vi "Close.vi"(8 "error in":errorcluster, 11 "IMAQdx Triggered Continuous Acquisition in":refnum<class "IMAQdx Triggered Continuous Acquisition.lvclass">) -> (0 "error out":errorcluster, 3 "IMAQdx Triggered Continuous Acquisition out":refnum<class "IMAQdx Triggered Continuous Acquisition.lvclass">)   [LabVIEW 2024, in "IMAQdx Triggered Continuous Acquisition.lvclass"]
uses:
  IMAQdx Triggered Continuous Acquisition.lvclass
  IMAQdx Triggered Continuous Acquisition.lvclass/IMAQdx Triggered Continuous Acquisition.ctl
  Base/IMAQdx Base Configure Strategy.lvclass
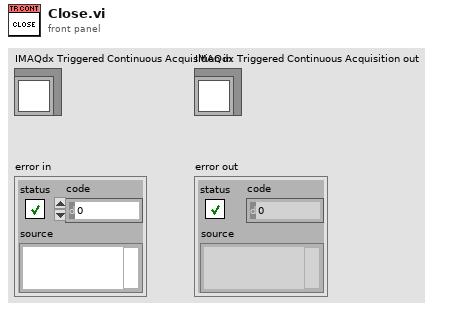
[diagram p1: front panel]
types:
  T1 = typedef "IMAQ Image.ctl" = refnum<image>
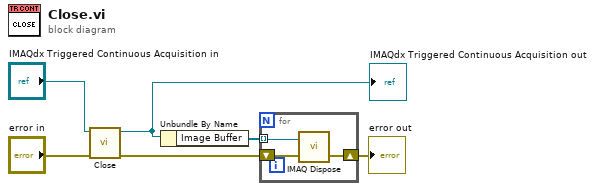
[diagram p0: block diagram]
diagram:
  n1 = call-parent "Close.vi"("error in"="error in", "IMAQdx Base Configure Strategy in"="IMAQdx Triggered Continuous Acquisition in") -> ("error out"=w3:errorcluster, "IMAQdx Base Configure Strategy out"=w4:refnum<class "IMAQdx Triggered Continuous Acquisition.lvclass">)  [unwired: 8 in]
  "IMAQdx Triggered Continuous Acquisition out" <- w4
  n2 = Unbundle By Name(w4) -> ("Image Buffer"=w1:T1[])
  n3 = for {
    shift-right: [w8] -> w2
    shift-left: w3 -> [w9]
    tunnel: w1 -> [w7] mode=indexing
    n4 = call "IMAQ Dispose"("Image"=w7, "error in (no error)"=w9) -> ("error out"=w8:errorcluster)  [unwired: 4 in]
  }
  "error out" <- w2
